vi "IR read.vi"(8 "error in (no error)":errorcluster, 11 "IR sensor in":refnum<class "IR sensor.lvclass">) -> (0 "error out":errorcluster, 2 "IR":dbl, 3 "IR sensor out":refnum<class "IR sensor.lvclass">)   [LabVIEW 2019, in "my FPGA lib.lvlib" / "IR sensor.lvclass"]
uses:
  IR sensor.lvclass
  IR sensor.lvclass/IR sensor.ctl
  <vilib>/Utility/error.llb/Error Cluster From Error Code.vi
  <vilib>/rvi/errors/niLvFpgaAdjustHostInterfaceError.vi
  <vilib>/rvi/interface/nirviReadWriteControl/nirviReadWriteControl.xnode
  FPGA/FPPGA.ctl
  NiFpgaLv.dll
  <vilib>/rvi/interface/Simulation/niFpgaSimulationCallBeginRW.vi
  my FPGA lib.lvlib
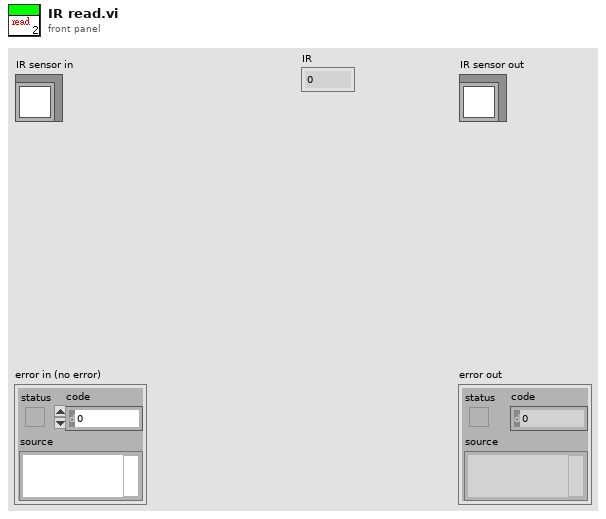
[diagram p1: front panel]
types:
  T1 = enum16{"IR.1", "IR.2", "IR.3", "IR.4", "IR.5", "IR.6", "IR.7", "IR.8"}
  T2 = typedef "my FPGA lib.lvlib/FPPGA.ctl" = refnum<k20>
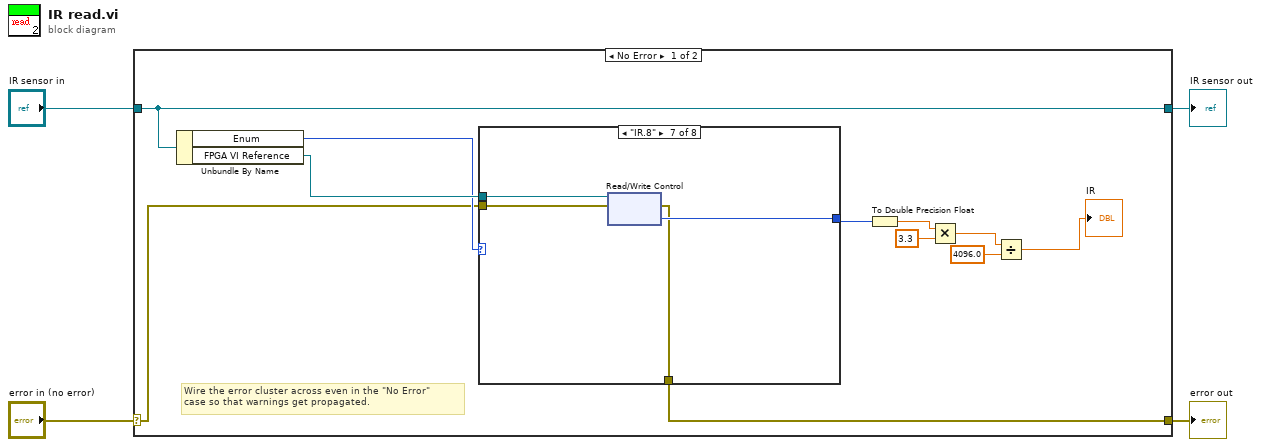
[diagram p0: block diagram]
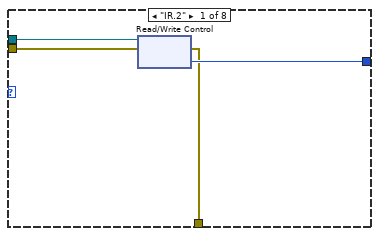
[diagram p2: hidden frame]
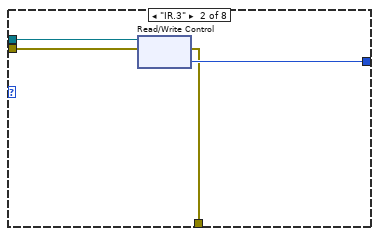
[diagram p3: hidden frame]
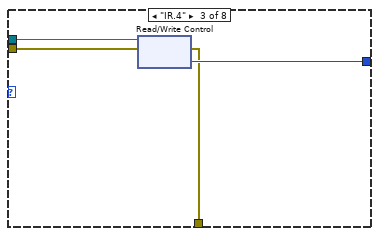
[diagram p4: hidden frame]
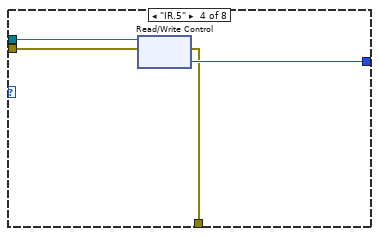
[diagram p5: hidden frame]
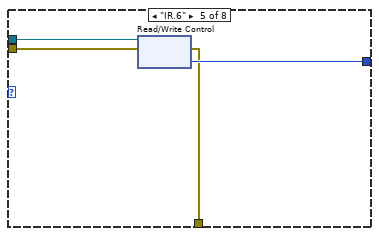
[diagram p6: hidden frame]
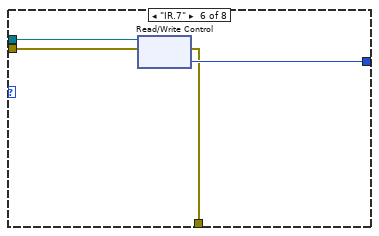
[diagram p7: hidden frame]
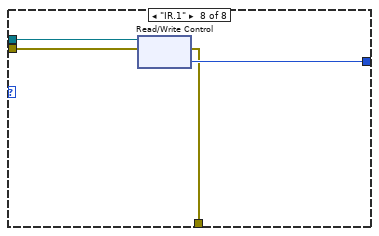
[diagram p8: hidden frame]
diagram:
  n1 = case shown="No Error" "error in (no error)" {
    selector: "error in (no error)" -> [w12 w49]
    tunnel: [w11 w49] -> w3
    tunnel: [w15 w48] -> w1
    tunnel: "IR sensor in" -> [w15 w48]
    frame No Error {
      # "Wire the error cluster across even in the \"No Error\"\ncase so that warnings get propagated."
      n2 = Unbundle By Name(w15) -> ("Enum"=w13:T1, "FPGA VI Reference"=w14:T2)
      n3 = case shown="\"IR.8\"" w13 {
        tunnel: w14 -> [w19 w23 w27 w31 w35 w39 w43 w47]
        tunnel: w12 -> [w18 w22 w26 w30 w34 w38 w42 w46]
        tunnel: [w17 w21 w25 w29 w33 w37 w41 w45] -> w10
        tunnel: [w16 w20 w24 w28 w32 w36 w40 w44] -> w11
        frame "IR.2" {
          n4 = xnode "Read/Write Control"("FPGA VI Reference In"=w19, "error in"=w18) -> ("error out"=w16:errorcluster, "IR 2"=w17:u16)  [unwired: 1 out]
        }
        frame "IR.3" {
          n5 = xnode "Read/Write Control"("FPGA VI Reference In"=w23, "error in"=w22) -> ("error out"=w20:errorcluster, "IR 3"=w21:u16)  [unwired: 1 out]
        }
        frame "IR.4" {
          n6 = xnode "Read/Write Control"("FPGA VI Reference In"=w27, "error in"=w26) -> ("error out"=w24:errorcluster, "IR 4"=w25:u16)  [unwired: 1 out]
        }
        frame "IR.5" {
          n7 = xnode "Read/Write Control"("FPGA VI Reference In"=w31, "error in"=w30) -> ("error out"=w28:errorcluster, "IR 5"=w29:u16)  [unwired: 1 out]
        }
        frame "IR.6" {
          n8 = xnode "Read/Write Control"("FPGA VI Reference In"=w35, "error in"=w34) -> ("error out"=w32:errorcluster, "IR 6"=w33:u16)  [unwired: 1 out]
        }
        frame "IR.7" {
          n9 = xnode "Read/Write Control"("FPGA VI Reference In"=w39, "error in"=w38) -> ("error out"=w36:errorcluster, "IR 7"=w37:u16)  [unwired: 1 out]
        }
        frame "IR.8" {
          n10 = xnode "Read/Write Control"("FPGA VI Reference In"=w43, "error in"=w42) -> ("error out"=w40:errorcluster, "IR 8"=w41:u16)  [unwired: 1 out]
        }
        frame "IR.1" {
          n11 = xnode "Read/Write Control"("FPGA VI Reference In"=w47, "error in"=w46) -> ("error out"=w44:errorcluster, "IR 1"=w45:u16)  [unwired: 1 out]
        }
      }
      n12 = To Double Precision Float(number=w10) -> (double precision float=w9:dbl)
      n13 = Multiply(x=w9, y=3.3) -> (x*y=w7:dbl)
      n14 = Divide(x=w7, y=4096.0) -> (x/y=→"IR":dbl)
    }
    frame Error {
    }
  }
  "error out" <- w3
  "IR sensor out" <- w1
